vi "PowerMeter Read.vi"(1 "错误输入（无错误）":errorcluster) -> (2 "功率计读数":string, 3 "错误输出":errorcluster, 4 "通信正常？":bool)   [LabVIEW 2018]
uses:
  <vilib>/Analysis/baseanly.llb/Mean (DBL).vi
  InOut/Reslut.vi
  <vilib>/Analysis/NI_AALBase.lvlib
panel:
  out "数组":dbl[](array[numeric])
  out "功率计输出":dbl
  out "Unit":string
  out "结果字符串":string
  out "数据输出":string
  # "通道B为功率计"
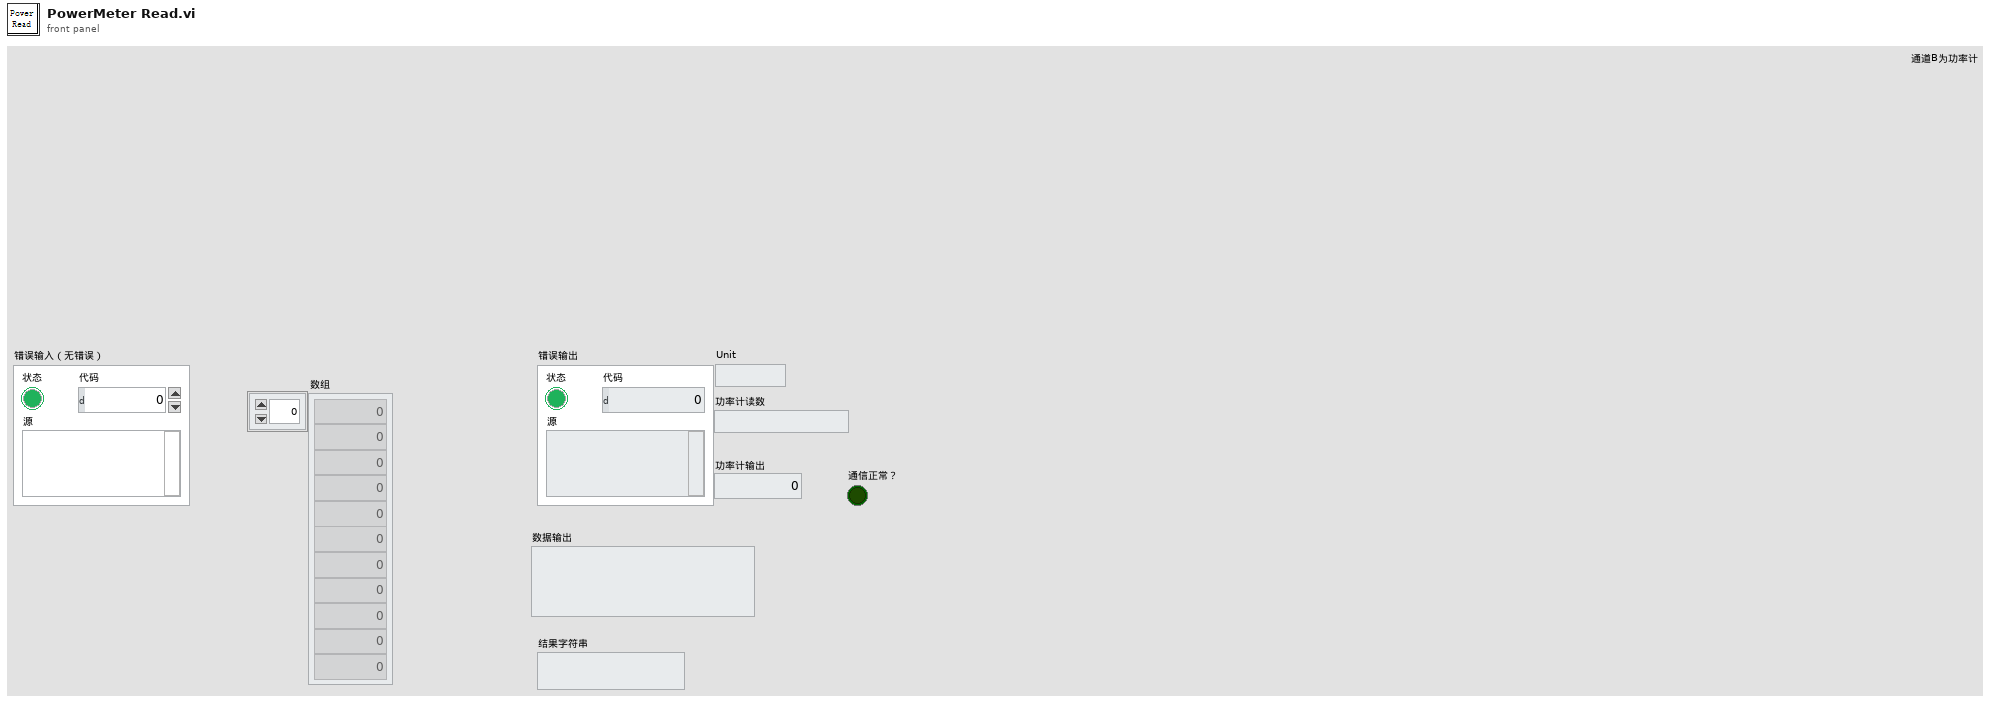
[diagram p1: front panel]
types:
  T1 = enum16{"Standard", "Buffered", "CRLF", "Immediate"}
  T2 = typedef "控制电机位置枚举器.ctl" = enum16{"远场扫描", "发散角扫描", "远场相机", "近场相机", "时间波形", "偏振", "能量", "功率", "光谱"}
  T3 = typedef "控制电机指令枚举器.ctl" = enum16{"归0", "停止", "运动", "轴设置", "通信连接"}
  T4 = typedef "控制电机枚举器.ctl" = enum16{"Z", "Y", "X", "发散角", "俯仰", "旋转"}
  T5 = typedef "IMAQ Image.ctl" = refnum<image>
  T6 = cluster{"示波器":cluster{"Channel (0:Channel 1)":enum16{"Channel 1", "Channel 2", "Channel 3", "Channel 4"}, "电压范围":dbl, "触发电压":dbl, "时间范围":dbl, " 示波器VISA":refnum<visa-resource-name>, "时间范围 标签":u64, "电压范围 标签":u64, "触发电压 标签":u64, "输入阻抗/Ω":u64}, "光谱仪":cluster{"SpecDataReference":refnum<queue>, "grating center":dbl, "Exposure Time (s)":dbl, "是否进行详细设置":bool, " 开始通信检查":bool, "通信成功？":bool, "波长":dbl}, " 近场相机":cluster{"曝光时间/100us":dbl, "模拟增益":i32, "控制套接字":i32, "IP 地址":string, " 采集套接字":i32, "  版本号":i32, "ImageData":T5, "  增益最大":i32, "  增益最小":i32, " 曝光最大":i32, " 曝光最小":i32, " 帧速":i32, " 同步切换":i32, "  曝光缩放":i32}, " 偏振仪":cluster{"电压范围":u64, "触发电压":u64, "时间范围":u64, "波长范围":enum16{"可见光 400-700nm", "近红外 700-1100nm"}, "可见光偏振测量仪VISA":refnum<visa-resource-name>, "近红外偏振测量仪VISA":refnum<visa-resource-name>}, " 功率计":cluster{"通道":enum16{"Channel 1", "Channel 2"}, "工作波长":u32, "单位":u64, "时间范围":u64, "IP地址":string, "端口":u32}, "能量计":cluster{"通道":enum16{"Channel 1", "Channel 2"}, "工作波长":u32, "单位":u64, "时间范围":u64, "IP地址":string, "端口":u32, "能量计量程":enum16{"200uJ", "20uJ", "2uJ", "200nJ"}}, "电机":cluster{"Channel (0:Channel 1)":enum16{"Channel 1", "Channel 2", "Channel 3", "Channel 4"}, "电压范围":u64, "触发电压":u64, "时间范围":u64}, " 远场相机":cluster{"曝光时间":i32, "模拟增益":i32, "控制套接字":i32, "IP 地址":string, " 采集套接字":i32, "  版本号":i32, "ImageData":T5, "  增益最大":i32, "  增益最小":i32, " 曝光最大":i32, " 曝光最小":i32, " 帧速":i32, " 同步切换":i32, "  曝光缩放":i32, "ImageData B":T5}}
  T7 = cluster{"能量计结果":string, "功率计结果":string, "能量计单位":string, " 功率计单位":string}
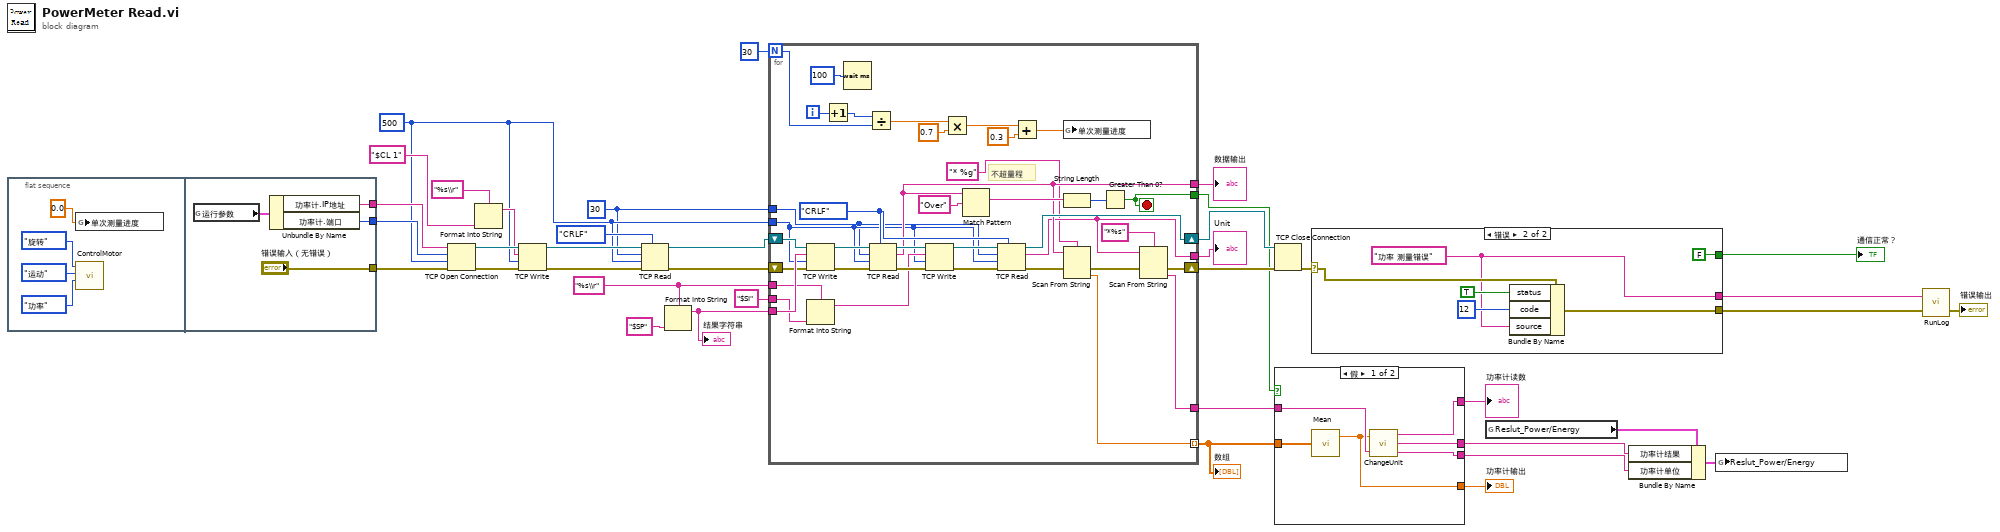
[diagram p0: block diagram]
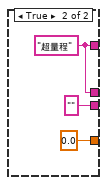
[diagram p2: hidden frame]
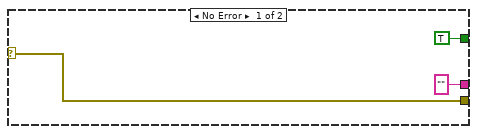
[diagram p3: hidden frame]
diagram:
  w11 = 30 ("读取的字节")
  w14 = 500 ("超时毫秒(25000)")
  w29 = "%s\\r" ("格式字符串")
  n1 = flat-sequence {
    tunnel: ["错误输入（无错误）"] -> w31
    tunnel: [w44] -> w27
    tunnel: [w43] -> w26
    frame #0 {
      n2 = global write "globalMessage.vi" "单次测量进度"(0.0 ("单次测量进度")) -> ()
      n3 = call "ControlMotor.vi"("控制电机"=控制电机枚举器."旋转", "控制电机指令"=控制电机指令枚举器."运动", "位置"=控制电机位置枚举器."功率") -> ()  [unwired: 5 in, 1 out]
    }
    frame #1 {
      n4 = global read "参数.vi" "运行参数"() -> (w45:T6)
      n5 = Unbundle By Name(w45) -> ("功率计.IP地址"=w44:string, "功率计.端口"=w43:u32)
    }
  }
  n6 = TCP Open Connection(address=w27, remote port or service name=w26, timeout ms (60000)=w14, error in (no error)=w31) -> (connection ID=w34:refnum<k5>, error out=w32:errorcluster)  [unwired: 1 in]
  n7 = Format Into String(format string="%s\\r" ("格式字符串"), "$CL 1" ("输入 1")) -> (resulting string=w33:string)  [unwired: 2 in, 1 out]
  n8 = TCP Write(connection ID=w34, data in=w33, error in (no error)=w32, 9:w14) -> (connection ID out=w17:refnum<k5>, error out=w13:errorcluster)  [unwired: 1 out]
  n9 = TCP Read(connection ID=w17, bytes to read=w11, error in (no error)=w13, 7:T1."CRLF" ("模式（标准）"), 9:w14) -> (connection ID out=w16:refnum<k5>, error out=w12:errorcluster)  [unwired: 1 out]
  n10 = Format Into String(format string=w29, "$SP" ("输入 1")) -> (resulting string=w37:string)  [unwired: 2 in, 1 out]
  "结果字符串" <- w37
  n11 = for {
    N: 30 -> [w53]
    tunnel: w37 -> [w84]
    tunnel: w29 -> [w79]
    tunnel: [w70] -> w25
    tunnel: [w69] -> w24
    tunnel: w14 -> [w66]
    tunnel: w11 -> [w64]
    tunnel: [w63] -> w8 mode=indexing
    shift-right: [w74] -> w28
    shift-left: w16 -> [w67]
    shift-right: [w47] -> w23
    shift-left: w12 -> [w65]
    tunnel: [w62] -> w7
    tunnel: [w59] -> w5
    tunnel: "$SI" ("输入 1") -> [w57]
    i -> [w54]
    stop <- w59 stop-if-true
    w77 = T1."CRLF" ("模式（标准）")
    # "不超量程"
    n12 = TCP Write(connection ID=w67, data in=w84, error in (no error)=w65, 9:w66) -> (connection ID out=w83:refnum<k5>, error out=w82:errorcluster)  [unwired: 1 out]
    n13 = Format Into String(format string=w79, w57) -> (resulting string=w78:string)  [unwired: 2 in, 1 out]
    n14 = Increment(x=w54) -> (x+1=w49:i32)
    n15 = Wait (ms)(milliseconds to wait=u32 100 ("等待时间（毫秒）")) -> ()  [unwired: 1 out]
    n16 = Divide(x=w49, y=w53) -> (x/y=w56:dbl)
    n17 = TCP Read(connection ID=w83, bytes to read=w64, error in (no error)=w82, 7:w77, 9:w66) -> (connection ID out=w81:refnum<k5>, data out=w70:string, error out=w80:errorcluster)
    n18 = TCP Write(connection ID=w81, data in=w78, error in (no error)=w80, 9:w66) -> (connection ID out=w76:refnum<k5>, error out=w75:errorcluster)  [unwired: 1 out]
    n19 = Multiply(x=w56, y=0.7) -> (x*y=w51:dbl)
    n20 = Match Pattern(string=w70, regular expression="Over" ("正则表达式")) -> (match substring=w72:string)  [unwired: 1 in, 3 out]
    n21 = TCP Read(connection ID=w76, bytes to read=w64, error in (no error)=w75, 7:w77, 9:w66) -> (connection ID out=w74:refnum<k5>, data out=w69:string, error out=w68:errorcluster)
    n22 = Add(x=w51, y=0.3) -> (x+y=w50:dbl)
    n23 = global write "globalMessage.vi" "单次测量进度"(w50) -> ()
    n24 = String Length(string=w72) -> (length=w71:i32)
    n25 = Scan From String(format string="* %g" ("格式字符串"), input string=w70, error in=w68) -> (error out=w48:errorcluster, output 1=w63:dbl)  [unwired: 2 in, 2 out]
    n26 = Greater Than 0?(x=w71) -> (x > 0?=w59:bool)
    n27 = Scan From String(format string="*%s" ("格式字符串"), input string=w69, error in=w48) -> (error out=w47:errorcluster, output 1=w62:string)  [unwired: 2 in, 2 out]
  }
  "数据输出" <- w25
  "Unit" <- w24
  "数组" <- w8
  n28 = TCP Close Connection(connection ID=w28, error in (no error)=w23) -> (error out=w30:errorcluster)  [unwired: 1 in, 1 out]
  n29 = case shown="假" w5 {
    tunnel: w8 -> [w90 _]
    tunnel: w7 -> [w89 _]
    tunnel: [w88 0.0] -> w6
    tunnel: [w87 w92] -> w4
    tunnel: [w86 "" ("UintOut")] -> w3
    tunnel: [w85 w92] -> w2
    frame False {
      n30 = call-poly <vilib>:"Mean.vi"("X"=w90) -> ("mean"=w88:dbl)  [unwired: 1 out]
      n31 = call "ChangeUnit.vi"("change in"=w88, "unit in"=w89) -> ("change out"=w85:string, "DataOut"=w87:string, "UintOut"=w86:string)
    }
    frame True {
      w92 = "超量程"
    }
  }
  "功率计读数" <- w2
  "功率计输出" <- w6
  n32 = case shown="错误" w30 {
    selector: w30 -> [w94 w101]
    tunnel: [TRUE FALSE] -> w22
    tunnel: [w94 w97] -> w21
    tunnel: ["" ("source") w98] -> w20
    frame No Error {
    }
    frame Error {
      w98 = "功率 测量错误" ("source")
      n33 = Bundle By Name(cluster=w101, "status"=TRUE, "code"=12, "source"=w98) -> (w97:errorcluster)
    }
  }
  "通信正常？" <- w22
  n34 = global read "Reslut.vi" "Reslut_Power/Energy"() -> (w10:T7)
  n35 = Bundle By Name(cluster=w10, "功率计结果"=w4, "功率计单位"=w3) -> (w18:T7)
  n36 = global write "Reslut.vi" "Reslut_Power/Energy"(w18) -> ()
  n37 = call "RunLog.vi"("error in"=w21, "Message"=w20) -> ("error out"=→"错误输出":errorcluster)  [unwired: 1 in]
